vi "QCA Generate Event.vi"(0 "Event Number":i32) -> ()   [LabVIEW 2019]
uses:
  QCA Global.vi
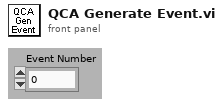
[diagram p1: front panel]
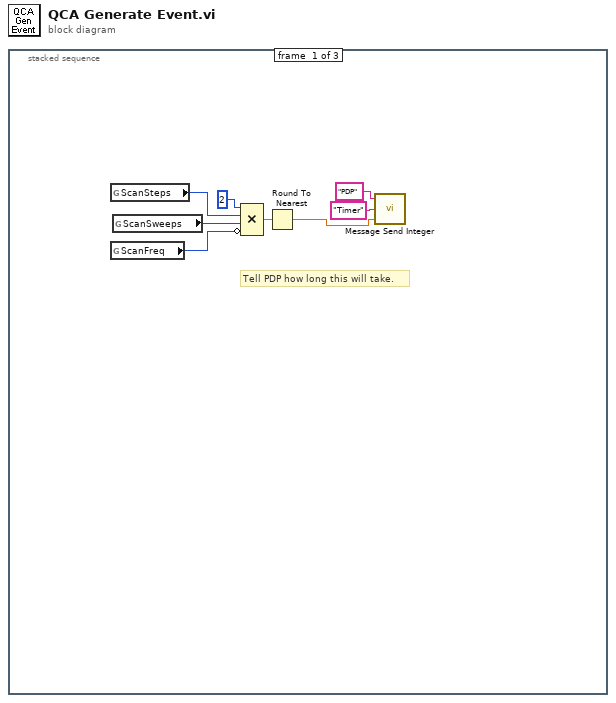
[diagram p0: block diagram]
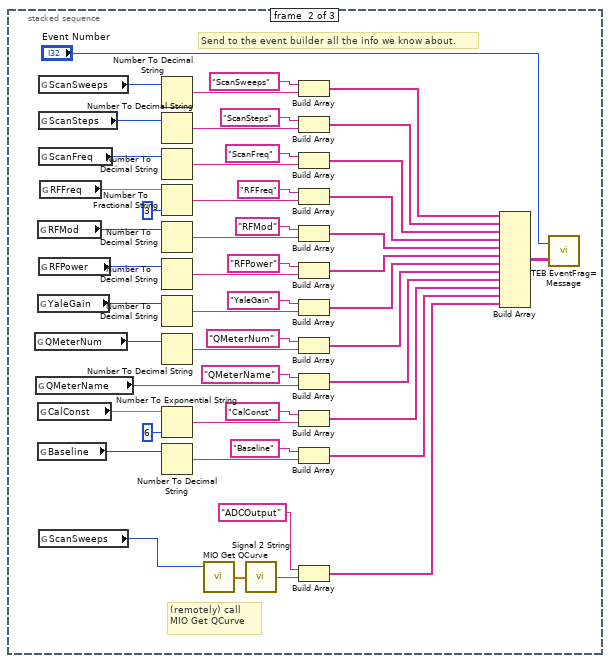
[diagram p2: hidden frame]
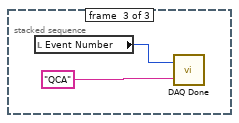
[diagram p3: hidden frame]
diagram:
  n1 = stacked-sequence {
    frame #0 {
      # "Tell PDP how long this will take."
      n2 = global read "QCA Global.vi" "ScanSteps"() -> (w2:i32)
      n3 = global read "QCA Global.vi" "ScanFreq"() -> (w4:i32)
      n4 = global read "QCA Global.vi" "ScanSweeps"() -> (w1:i32)
      n5 = Compound Arithmetic op=MULTIPLY(2 ("Input"), w2, w1, invert w4) -> (w5:dbl)
      n6 = Round To Nearest(number=w5) -> (nearest integer value=w8:dbl)
      n7 = call "Message Send Integer.vi"("Value"=w8, "Parameter"="Timer", "Destination"="PDP") -> ()
    }
    frame #1 {
      # "(remotely) call MIO Get QCurve"
      # "Send to the event builder all the info we know about."
      n8 = global read "QCA Global.vi" "QMeterNum"() -> (w18:i32)
      n9 = global read "QCA Global.vi" "QMeterName"() -> (w31:string)
      n10 = global read "QCA Global.vi" "RFMod"() -> (w47:i32)
      n11 = global read "QCA Global.vi" "YaleGain"() -> (w41:i32)
      n12 = global read "QCA Global.vi" "CalConst"() -> (w37:dbl)
      n13 = global read "QCA Global.vi" "Baseline"() -> (w32:i32)
      n14 = global read "QCA Global.vi" "ScanSweeps"() -> (w59:i32)
      n15 = global read "QCA Global.vi" "ScanSteps"() -> (w54:i32)
      n16 = global read "QCA Global.vi" "ScanFreq"() -> (w53:i32)
      n17 = global read "QCA Global.vi" "RFPower"() -> (w42:i32)
      n18 = global read "QCA Global.vi" "ScanSweeps"() -> (w9:i32)
      n19 = global read "QCA Global.vi" "RFFreq"() -> (w48:dbl)
      n20 = Number To Decimal String(number=w59) -> (decimal integer string=w58:string)  [unwired: 1 in]
      n21 = Number To Decimal String(number=w54) -> (decimal integer string=w55:string)  [unwired: 1 in]
      n22 = Number To Decimal String(number=w53) -> (decimal integer string=w52:string)  [unwired: 1 in]
      n23 = Number To Fractional String(number=w48, precision (6)=i16 3) -> (F-format string=w49:string)  [unwired: 2 in]
      n24 = Number To Decimal String(number=w47) -> (decimal integer string=w46:string)  [unwired: 1 in]
      n25 = Number To Decimal String(number=w42) -> (decimal integer string=w43:string)  [unwired: 1 in]
      n26 = Number To Decimal String(number=w41) -> (decimal integer string=w40:string)  [unwired: 1 in]
      n27 = Number To Decimal String(number=w18) -> (decimal integer string=w19:string)  [unwired: 1 in]
      n28 = Number To Exponential String(number=w37, precision (6)=i16 6) -> (E-format string=w36:string)  [unwired: 2 in]
      n29 = Number To Decimal String(number=w32) -> (decimal integer string=w33:string)  [unwired: 1 in]
      n30 = call "MIO Get QCurve.vi"("Num Sweeps"=w9) -> ("Waveform Graph"=w10:dbl[])  [unwired: 2 in]
      n31 = call "Signal 2 String.vi"("Signal"=w10) -> ("String"=w11:string)
      n32 = Build Array("ScanSweeps" ("Substring"), w58) -> (w28:string[])
      n33 = Build Array("ScanSteps" ("Substring"), w55) -> (w27:string[])
      n34 = Build Array("ScanFreq" ("Substring"), w52) -> (w26:string[])
      n35 = Build Array("RFFreq" ("Substring"), w49) -> (w25:string[])
      n36 = Build Array("RFMod" ("Substring"), w46) -> (w22:string[])
      n37 = Build Array("RFPower" ("Substring"), w43) -> (w23:string[])
      n38 = Build Array("YaleGain" ("Substring"), w40) -> (w24:string[])
      n39 = Build Array("QMeterNum" ("Substring"), w19) -> (w14:string[])
      n40 = Build Array("QMeterName" ("Substring"), w31) -> (w15:string[])
      n41 = Build Array("CalConst" ("Substring"), w36) -> (w16:string[])
      n42 = Build Array("Baseline" ("Substring"), w33) -> (w17:string[])
      n43 = Build Array("ADCOutput", w11) -> (w13:string[])
      n44 = Build Array(w28, w27, w26, w25, w22, w23, w24, w14, w15, w16, w17, w13) -> (w21:string[][])
      n45 = call "TEB EventFrag= Message.vi"("Event Fragment(s)"=w21, "Event Number"="Event Number") -> ()
    }
    frame #2 {
      n46 = local read "Event Number"() -> (w62:i32)
      n47 = call "DAQ Done.vi"("Module Name"="QCA", "Event Number"=w62) -> ()
    }
  }
